vi "ReadData.vi"(8 "Error In":errorcluster, 11 "File Path Control":path) -> (0 "Error Out":errorcluster, 1 "Y":dbl[](array[numeric]), 2 "X":dbl[](array[numeric]), 3 "File Path Control out":path)   [LabVIEW 2015]
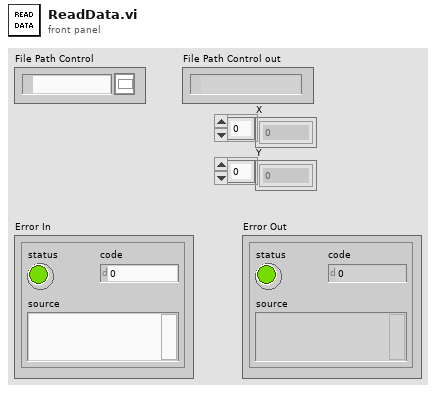
[diagram p1: front panel]
types:
  T1 = enum16{"open", "replace", "create", "open or create", "replace or create", "replace or create with confirmation"}
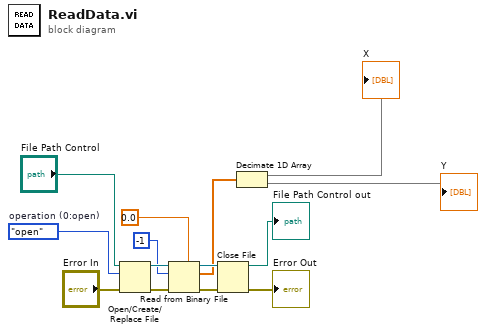
[diagram p0: block diagram]
diagram:
  w13 = T1."open"  # operation (0:open)
  n1 = Open/Create/Replace File(file path (use dialog)="File Path Control", error in="Error In", operation (0:open)=w13) -> (refnum out=w6:refnum<file>, error out=w7:errorcluster)  [unwired: 3 in, 1 out]
  n2 = Read from Binary File(5:0.0 ("element"), 8:w7, 10:-1 ("count (1)"), 11:w6) -> (0:w11:errorcluster, 2:w3:dbl[], 3:w9:refnum<file>)  [unwired: 2 in, 1 out]
  n3 = Close File(refnum=w9, error in=w11) -> (path=→"File Path Control out":path, error out=→"Error Out":errorcluster)
  n4 = Decimate 1D Array(w3) -> (→"X":dbl[], →"Y":dbl[])
